vi "Get total frames.vi"(11 "Acquisition cluster":T1 {"Cropping"."Height" min=0 max=2054 step=1; "Cropping"."Width" min=256 max=2456 step=8; "Cropping"."PosX Blue" min=0 max=2200 step=1; "Cropping"."PosY Blue" min=-2 max=1798 step=1; "Cropping"."PosX Green" min=0 max=1944 step=1; "Cropping"."PosY Green" min=-2 max=1542 step=1; "Cropping"."PosX Red" min=0 max=1944 step=1; "Cropping"."PosY Red" min=-2 max=1542 step=1}) -> (3 "Numeric":i32)   [LabVIEW 2017]
uses:
  Acquisition cluster.ctl
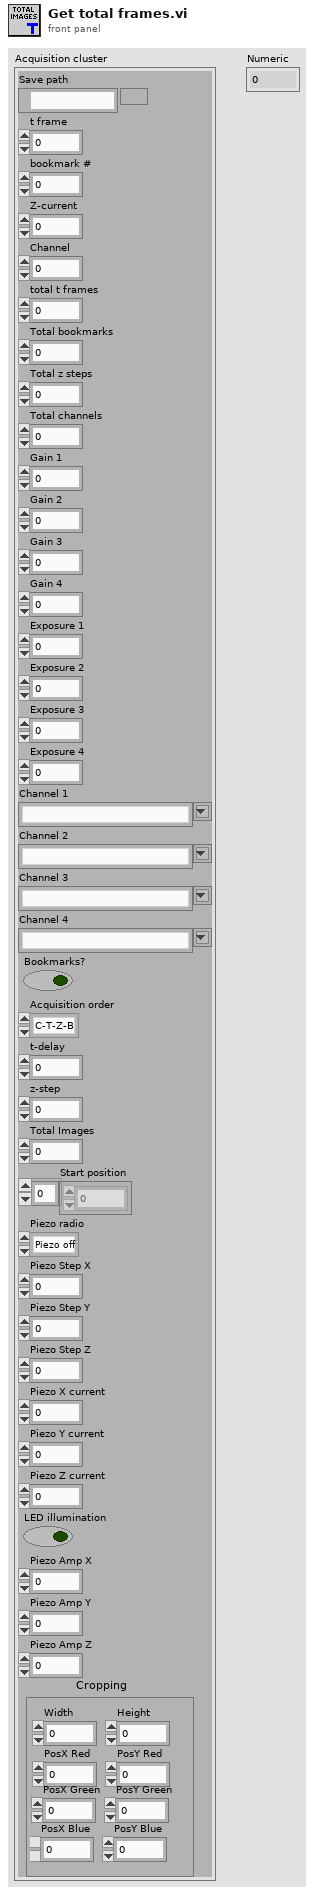
[diagram p1: front panel]
types:
  T1 = typedef "Acquisition cluster.ctl" = cluster{"Save path":path, "t frame":i32, "bookmark #":i32, "Z-current":i32, "Channel":i32, "total t frames":i32, "Total bookmarks":i32, "Total z steps":i32, "Total channels":i32, "Gain 1":i32, "Gain 2":i32, "Gain 3":i32, "Gain 4":i32, "Exposure 1":dbl, "Exposure 2":dbl, "Exposure 3":dbl, "Exposure 4":dbl, "Channel 1":string, "Channel 2":string, "Channel 3":string, "Channel 4":string, "Bookmarks?":bool, "Acquisition order":enum16{"C-T-Z-B", "C-T-B-Z", "C-Z-T-B", "C-Z-B-T", "C-B-T-Z", "C-B-Z-T", "T-C-Z-B", "T-C-B-Z", "T-Z-C-B", "T-Z-B-C", "T-B-C-Z", "T-B-Z-C", "Z-C-T-B", "Z-C-B-T", "Z-T-C-B", "Z-T-B-C", "Z-B-C-T", "Z-B-T-C", "B-C-T-Z", "B-C-Z-T", "B-Z-C-T", "B-Z-T-C", "B-T-C-Z", "B-T-Z-C"}, "t-delay":dbl, "z-step":dbl, "Total Images":i32, "Start position":dbl[], "Piezo radio":enum32{"Piezo off", "Piezo wiggle", "Piezo step"}, "Piezo Step X":dbl, "Piezo Step Y":dbl, "Piezo Step Z":dbl, "Piezo X current":dbl, "Piezo Y current":dbl, "Piezo Z current":dbl, "LED illumination":bool, "Piezo Amp X":dbl, "Piezo Amp Y":dbl, "Piezo Amp Z":dbl, "Cropping":cluster{"PosX Red":i32, "PosY Red":i32, "PosX Green":i32, "PosY Green":i32, "PosX Blue":i32, "PosY Blue":i32, "Width":i32, "Height":i32}}
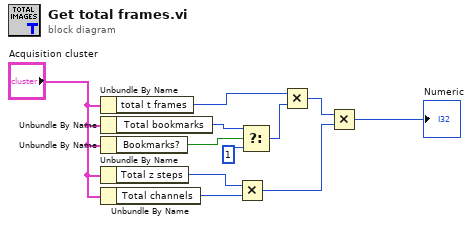
[diagram p0: block diagram]
diagram:
  n1 = Unbundle By Name("Acquisition cluster") -> ("total t frames"=w1:i32)
  n2 = Unbundle By Name("Acquisition cluster") -> ("Total bookmarks"=w7:i32)
  n3 = Unbundle By Name("Acquisition cluster") -> ("Bookmarks?"=w9:bool)
  n4 = Unbundle By Name("Acquisition cluster") -> ("Total z steps"=w2:i32)
  n5 = Unbundle By Name("Acquisition cluster") -> ("Total channels"=w3:i32)
  n6 = Multiply(x=w2, y=w3) -> (x*y=w5:i32)
  n7 = Select(t=w7, s=w9, f=1) -> (s? t:f=w10:i32)
  n8 = Multiply(x=w1, y=w10) -> (x*y=w6:i32)
  n9 = Multiply(x=w6, y=w5) -> (x*y=→"Numeric":i32)
